vi "MEASURE_2dmapping-2.vi"() -> ()   [LabVIEW 2020]
uses:
  <vilib>/Math Plots/3D Math Plots/3D Surface/3D Surface XCtrl/3D Surface.xctl
  <vilib>/Math Plots/3D Math Plots/3D Surface/3D Surface Datatype/3D Surface Datatype.lvclass
  <instrlib>/Keithley 24XX/Public/Data/Read (Multiple Points).vi
  <vilib>/Utility/file.llb/Write To Spreadsheet File (DBL).vi
  <vilib>/Math Plots/3D Math Plots/3D Surface/3D Surface Datatype/Public/Plot Helper (Vector).vi
  C/Program Files/National Instruments/LabVIEW 2016/instr.lib/Stanford Research 830/Stanford Research 830.lvlib
  C/Program Files/National Instruments/LabVIEW 2016/instr.lib/Keithley 2450/Keithley 2450.lvlib
  <instrlib>/Keithley 24XX/Keithley 24XX.lvlib
  <vilib>/Analysis/NI_AALBase.lvlib
panel:
  in  "GATE / SD stablization 5":dbl=0.1 format="%#_13g"
  in  "GATE / SD stablization 4":dbl=0.1 format="%#_13g"
  in  "ramping step":i32=20
  in  "Compliance  Level (1uA) 2":dbl=1e-08
  in  "Source Mode  (0: Voltage) 2":u16(ring) items=["Voltage", "Current"]
  out "3D Surface":refnum<class "3D Plot Datatype.lvclass">[](xcontrol)
  in  "scaning step2":i32=60
  out "gate voltage1":dbl=3.0 format="%#_13g"
  in  "scanning step1":i32=30
  in  "GATE2 end Value   2":dbl=10.0
  in  "GATE2 starting Value  2":dbl=-14.0
  out "gate 2leaking":dbl=1.1399661770106206e-10
  out "gate voltage2":dbl=10.0 format="%#_13g"
  in  "Serial Configuration":T1={"Baud Rate"=9600, "Parity"=0, "Data Bits"=8, "Stop Bits"=10, "Flow Control"=0} {"Flow Control" items=["None", "XON/XOFF", "RTS/CTS", "XON/XOFF & RTS/CTS", "DTR/DSR", "XON/XOFF & DTR/DSR"]; "Stop Bits" items=["1.0"=10, "1.5"=15, "2.0"=20]; "Data Bits" items=["7"=7, "8"=8]; "Parity" items=["None", "Odd", "Even", "Mark", "Space"]; "Baud Rate" items=["300"=300, "600"=600, "1200"=1200, "2400"=2400, "4800"=4800, "9600"=9600, "19200"=19200]}
  in  "gate2 address":refnum<visa-resource-name>="GPIB0::25::INSTR"
  in  "Save data or not":bool=TRUE
  in  "path (folder + filename)":string="C:\\Users\\User\\Data\\Jason\\03282019\\mapping_3"
  out "XY Graph":cluster{dbl[], dbl[]}(graph)={[-14.0, -13.6, -13.2, -12.8, -12.4, -12.0, -11.6, -11.2, -10.8, -10.4, -10.0, -9.6, -9.2, -8.8, -8.399999999999999, -8.0, -7.6, -7.199999999999999, -6.8, -6.3999999999999995, -6.0, -5.6, -5.199999999999999, -4.799999999999999, -4.399999999999999, -4.0, -3.5999999999999996, -3.1999999999999993, -2.799999999999999, -2.3999999999999986, -2.0, -1.5999999999999996, -1.1999999999999993, -0.7999999999999989, -0.3999999999999986, 0.0, 0.40000000000000036, 0.8000000000000007, 1.200000000000001, 1.6000000000000014, 2.0, 2.400000000000002, 2.8000000000000007, 3.1999999999999993, 3.6000000000000014, 4.0, 4.400000000000002, 4.800000000000001, 5.200000000000003, 5.600000000000001, 6.0, 6.400000000000002, 6.800000000000001, 7.200000000000003, 7.600000000000001, 8.0, 8.400000000000002, 8.8, 9.200000000000003, 9.600000000000001, 10.0], [0.000948314, 0.000947837, 0.000947598, 0.000947479, 0.000947241, 0.000946883, 0.000946645, 0.000945572, 0.000944141, 0.000942711, 0.000941519, 0.000939969, 0.000938658, 0.000937108, 0.00093532, 0.000933651, 0.000931863, 0.000929955, 0.000928048, 0.000926021, 0.000923995, 0.00092173, 0.000919465, 0.0009172, 0.000914697, 0.000912312, 0.000909809, 0.000907306, 0.000904683, 0.00090218, 0.000899557, 0.000896934, 0.000894193, 0.00089157, 0.000888947, 0.000886325, 0.000883702, 0.00088108, 0.000878457, 0.000875834, 0.000873331, 0.000870828, 0.000868324, 0.00086594, 0.000863437, 0.000861172, 0.000858787, 0.000856522, 0.000854257, 0.000852112, 0.000849966, 0.000847939, 0.000846032, 0.000844125, 0.000842217, 0.000840429, 0.000838879, 0.000837211, 0.000835661, 0.00083435, 0.000833277]}
  out "LOCKIN Measurement":dbl=0.000833277
  in  "Parameter (1: X)":u16(ring)=1 items=["X"=1, "Y"=2, "R"=3, "Theta"=4, "Channel 1"=5, "Channel 2"=6, "Aux In 1"=7, "Aux In 2"=8, "Aux In 3"=9, "Aux In 4"=10]
  out "gate leaking":string="4.458176E-12\n"
  in  "GATE1 end Value (default 0)":dbl=3.0
  in  "GATE1 starting(small) Value":dbl=-3.0
  in  "Function (0: Volts) 2":u16(ring) items=["Volts", "Current", "Resistance"]
  in  "Source Compaliance":dbl=1e-08
  in  "gate1 address":refnum<visa-resource-name>="GPIB0::18::INSTR"
  in  "SD stabilization(S) 2":dbl=0.1 format="%#_13g"
  in  "Sine Output Amplitude (1 V) 2":dbl=0.05
  in  "GATE / SD stablization 3":dbl=0.2 format="%#_13g"
  in  "frequency":dbl=50.0 format="%#_13g"
  in  "Input Connection (0: Single-Ended Voltage)":u16(ring) items=["Single-Ended Voltage", "Differential Voltage", "1 MOhm Current Gain", "100 MOhm Current Gain"]
  in  "LOCKIN address":refnum<visa-resource-name>="GPIB0::8::INSTR"
  # "Lock-in"
  # "2450 Gate Setting"
  # "2401 Gate Setting"
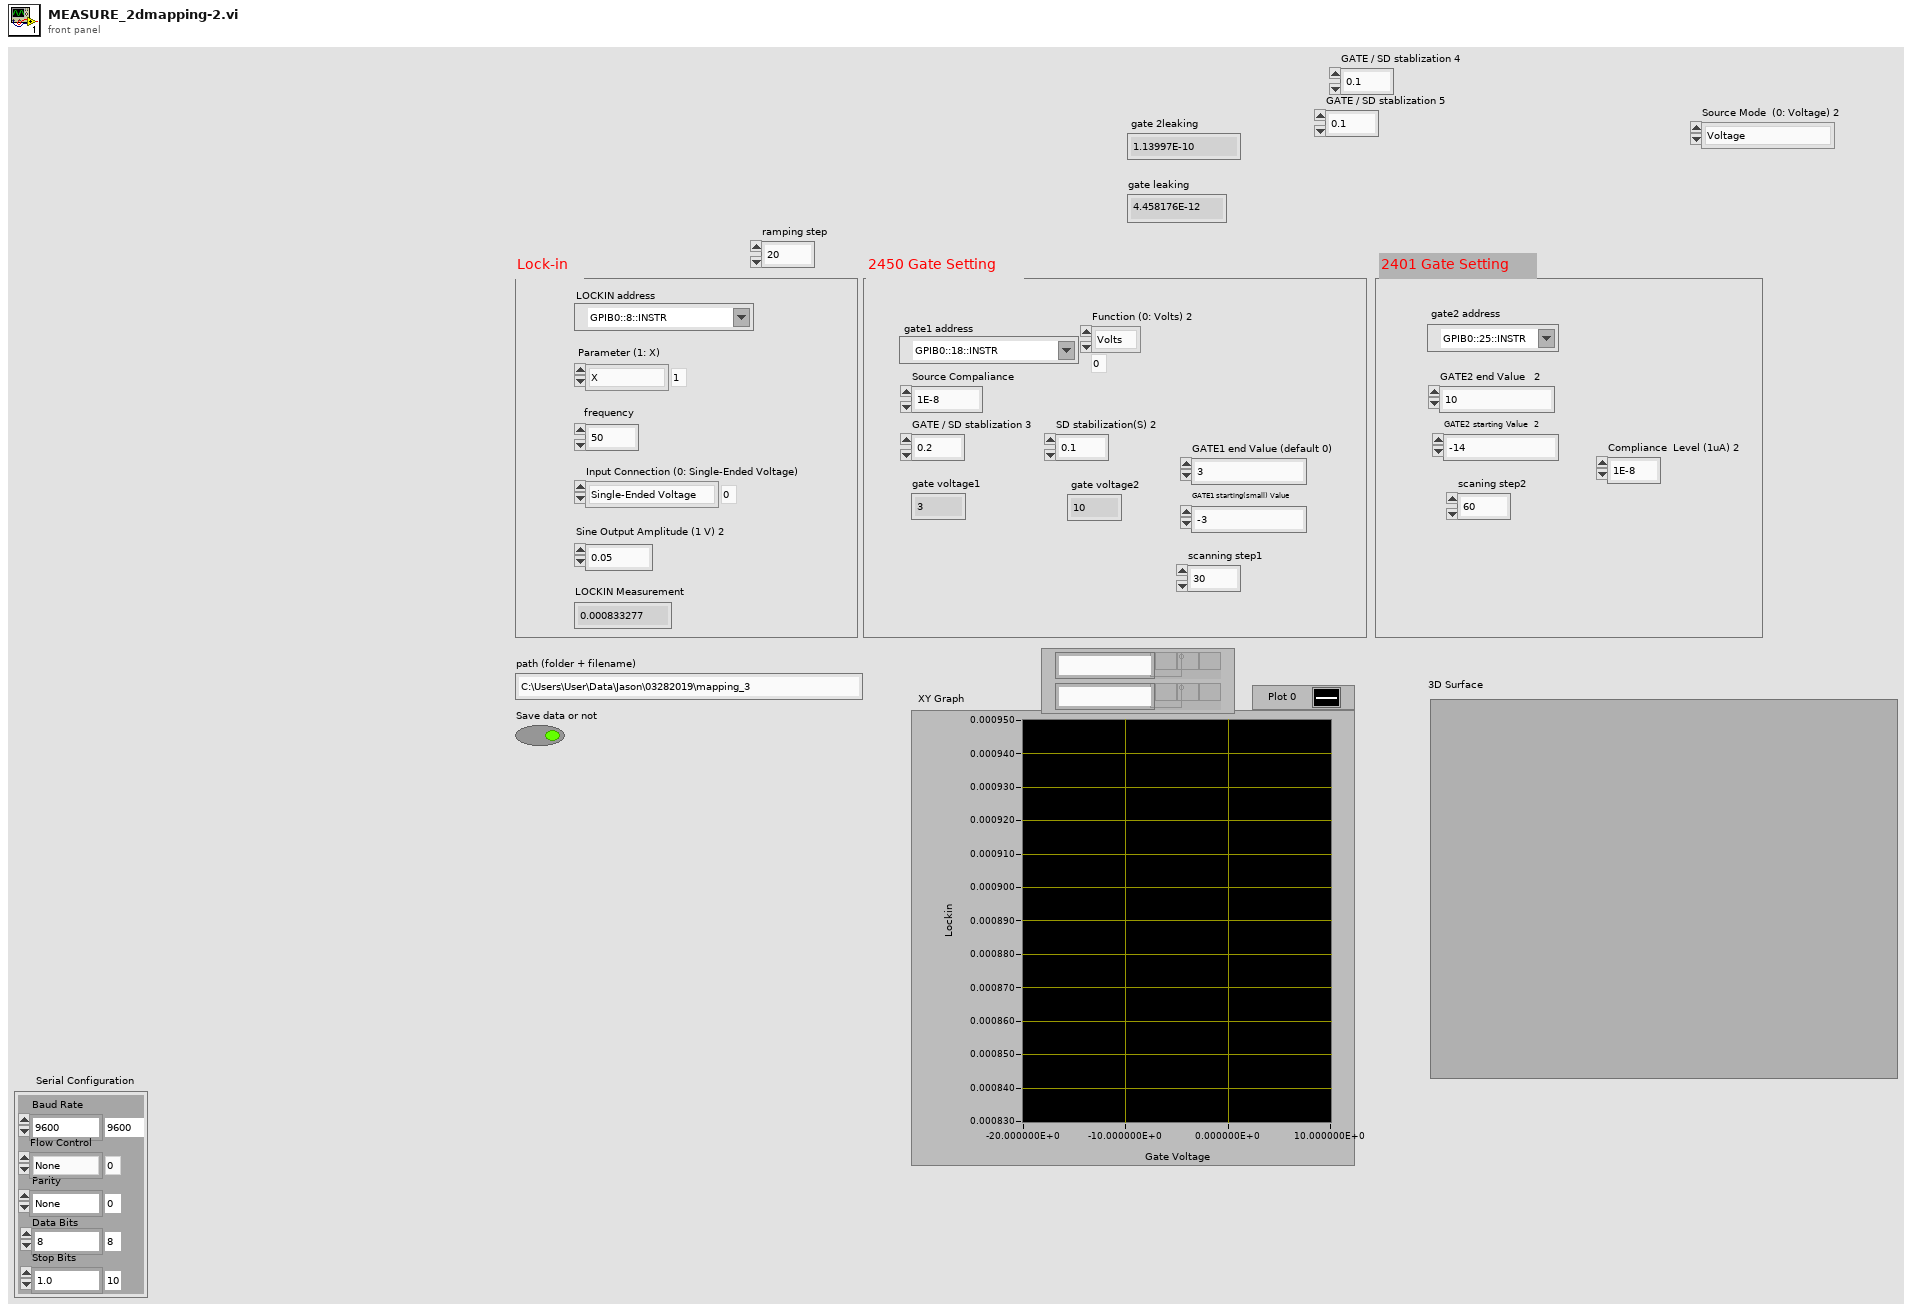
[diagram p1: front panel]
types:
  T1 = cluster{"Baud Rate":u32, "Parity":u16, "Data Bits":u16, "Stop Bits":u16, "Flow Control":u16}
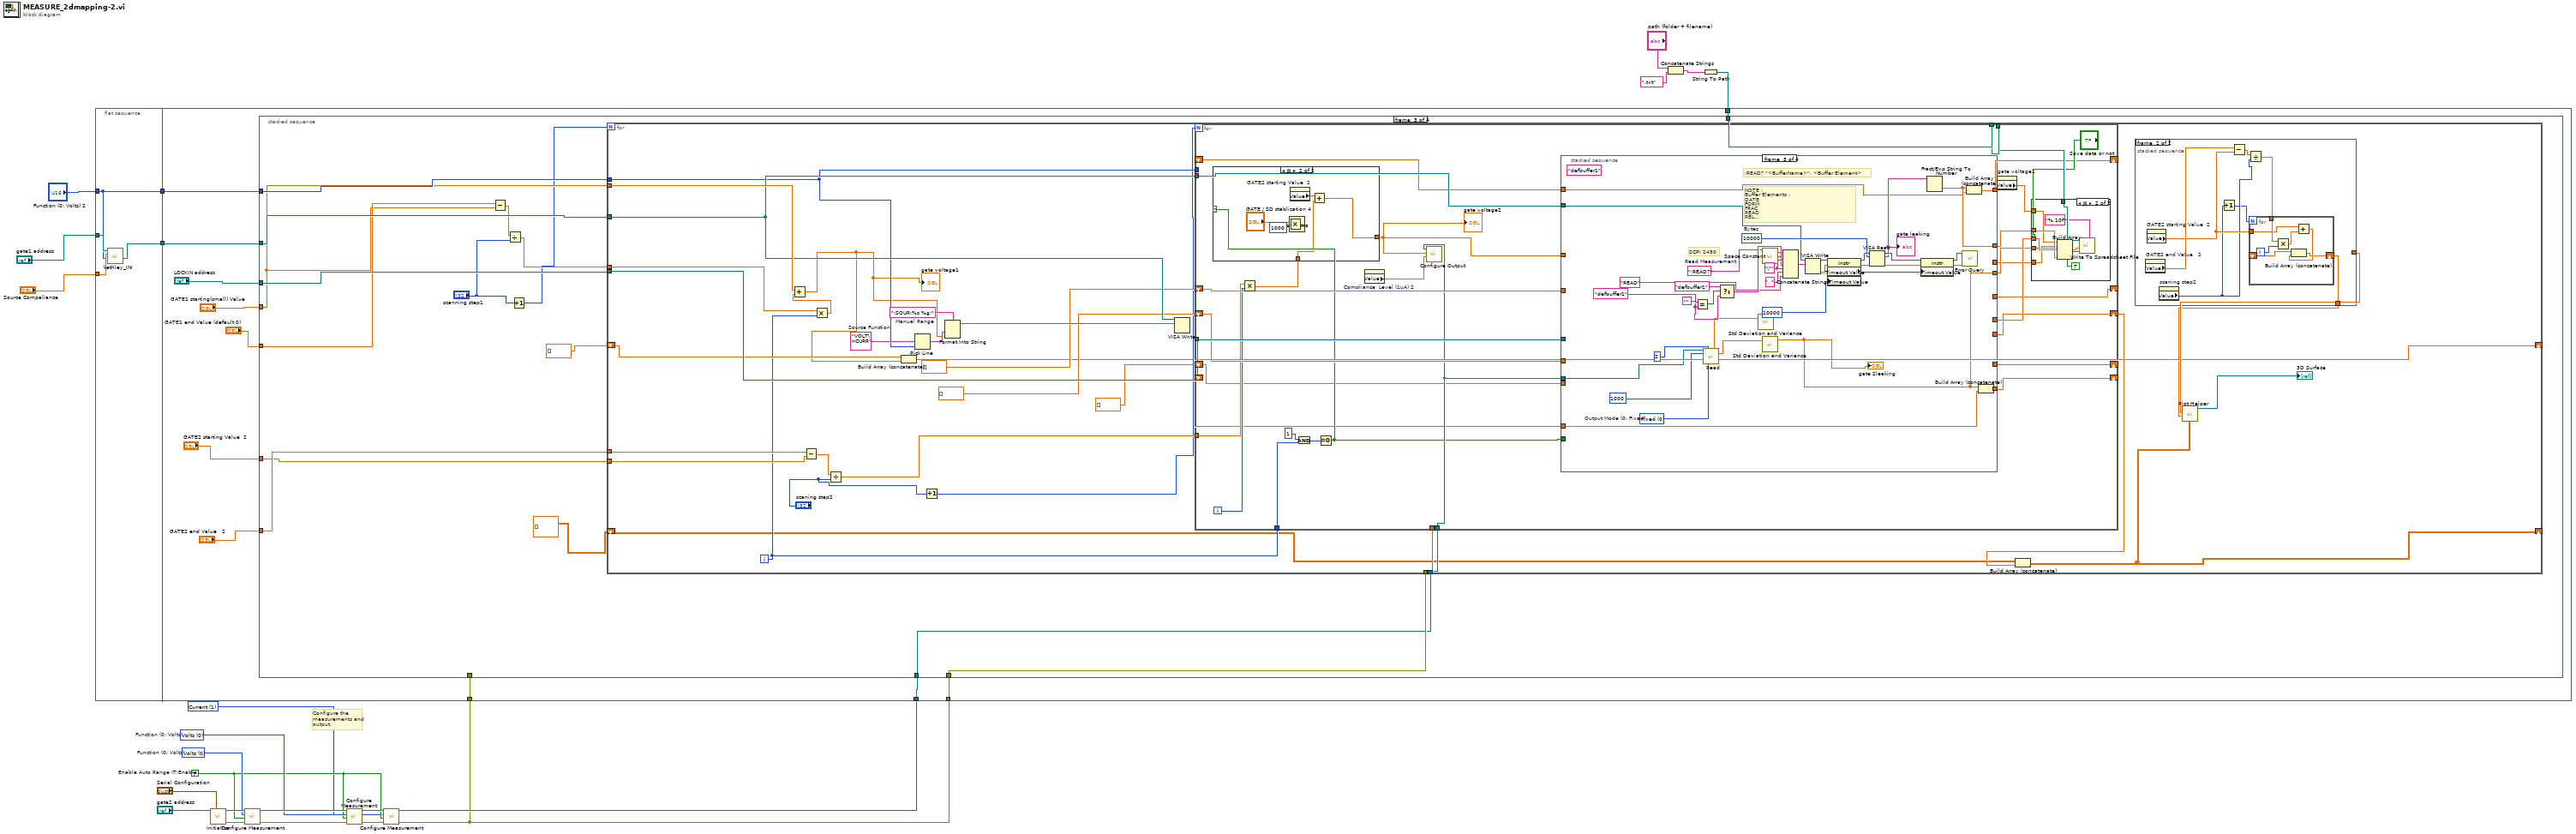
[diagram p0: block diagram]
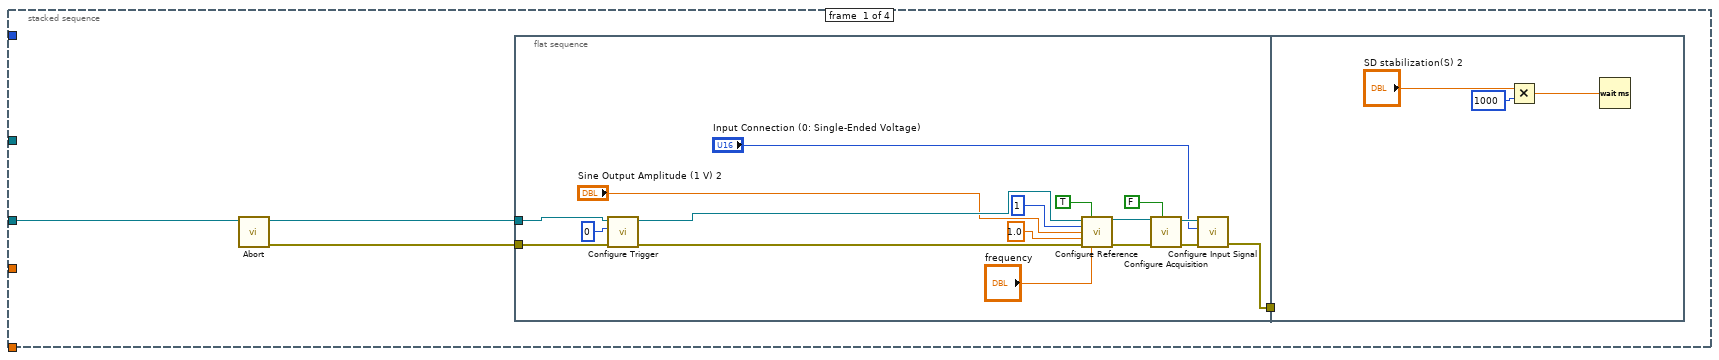
[diagram p2: hidden frame]
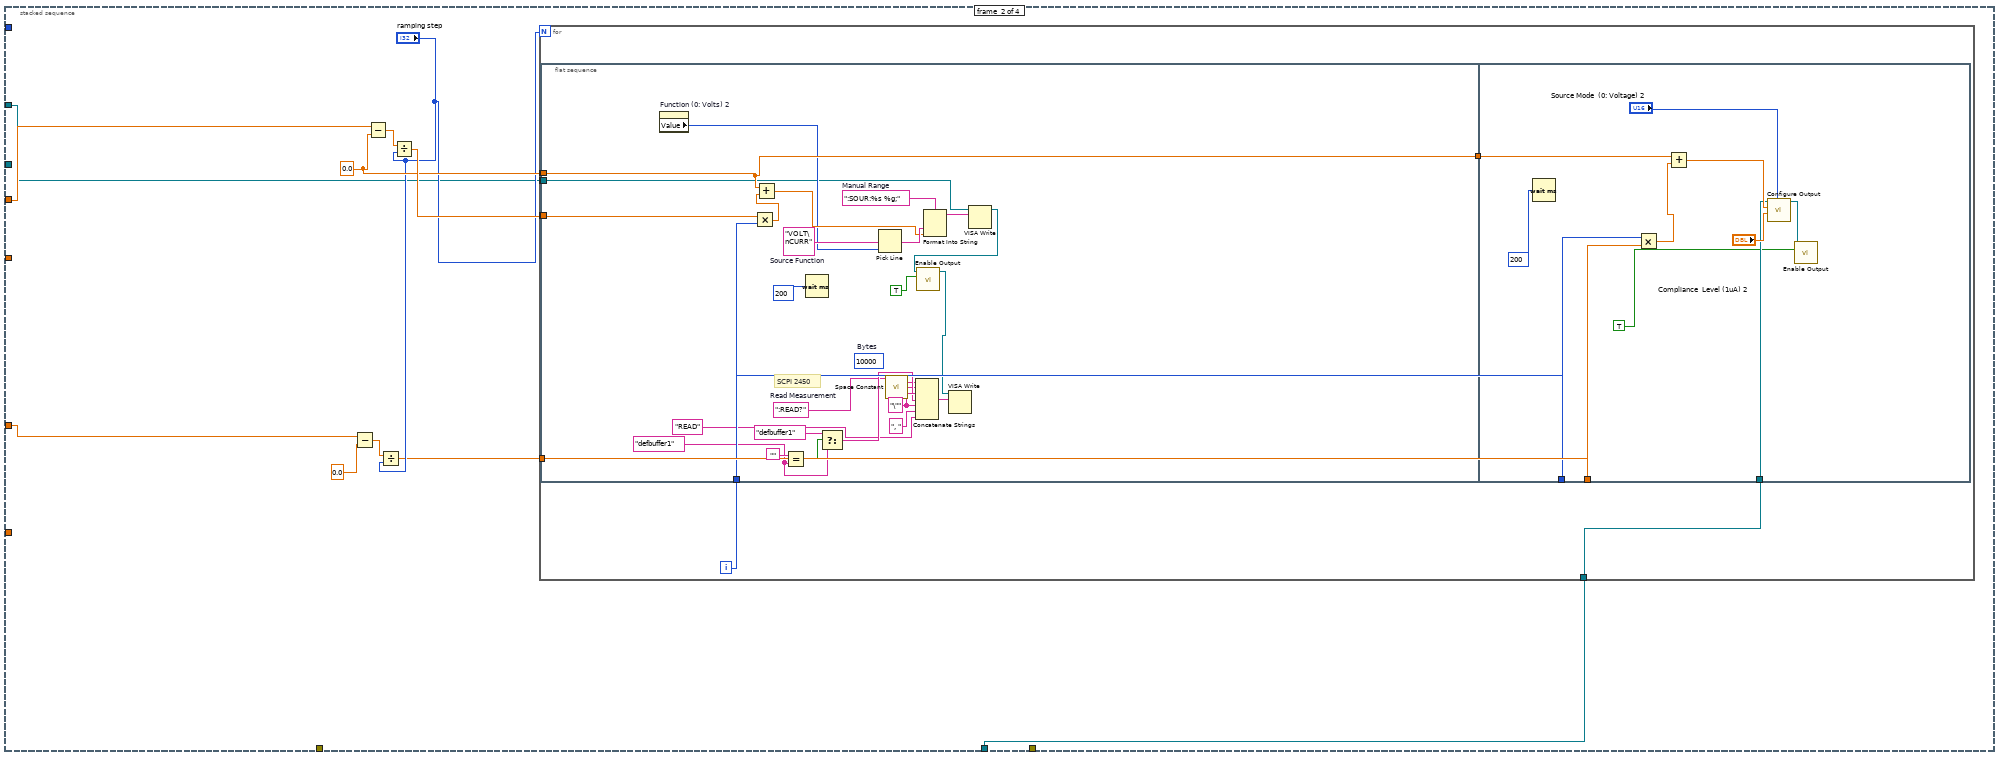
[diagram p3: hidden frame]
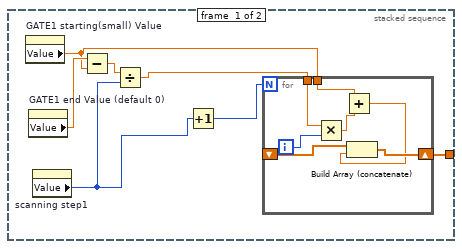
[diagram p4: hidden frame]
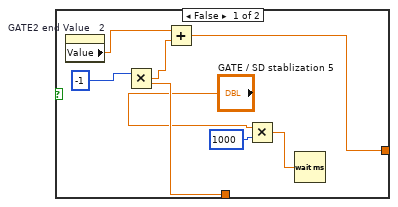
[diagram p5: hidden frame]
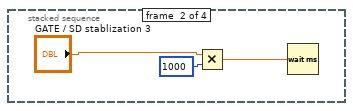
[diagram p8: hidden frame]
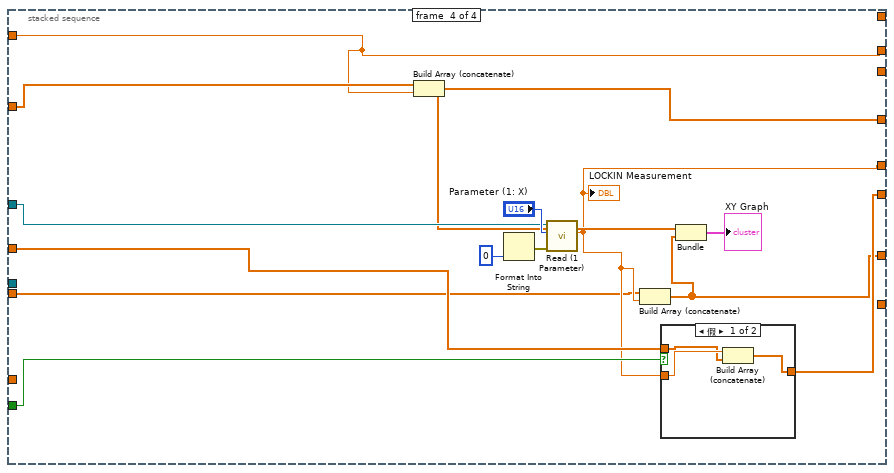
[diagram p9: hidden frame]
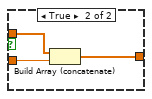
[diagram p10: hidden frame]
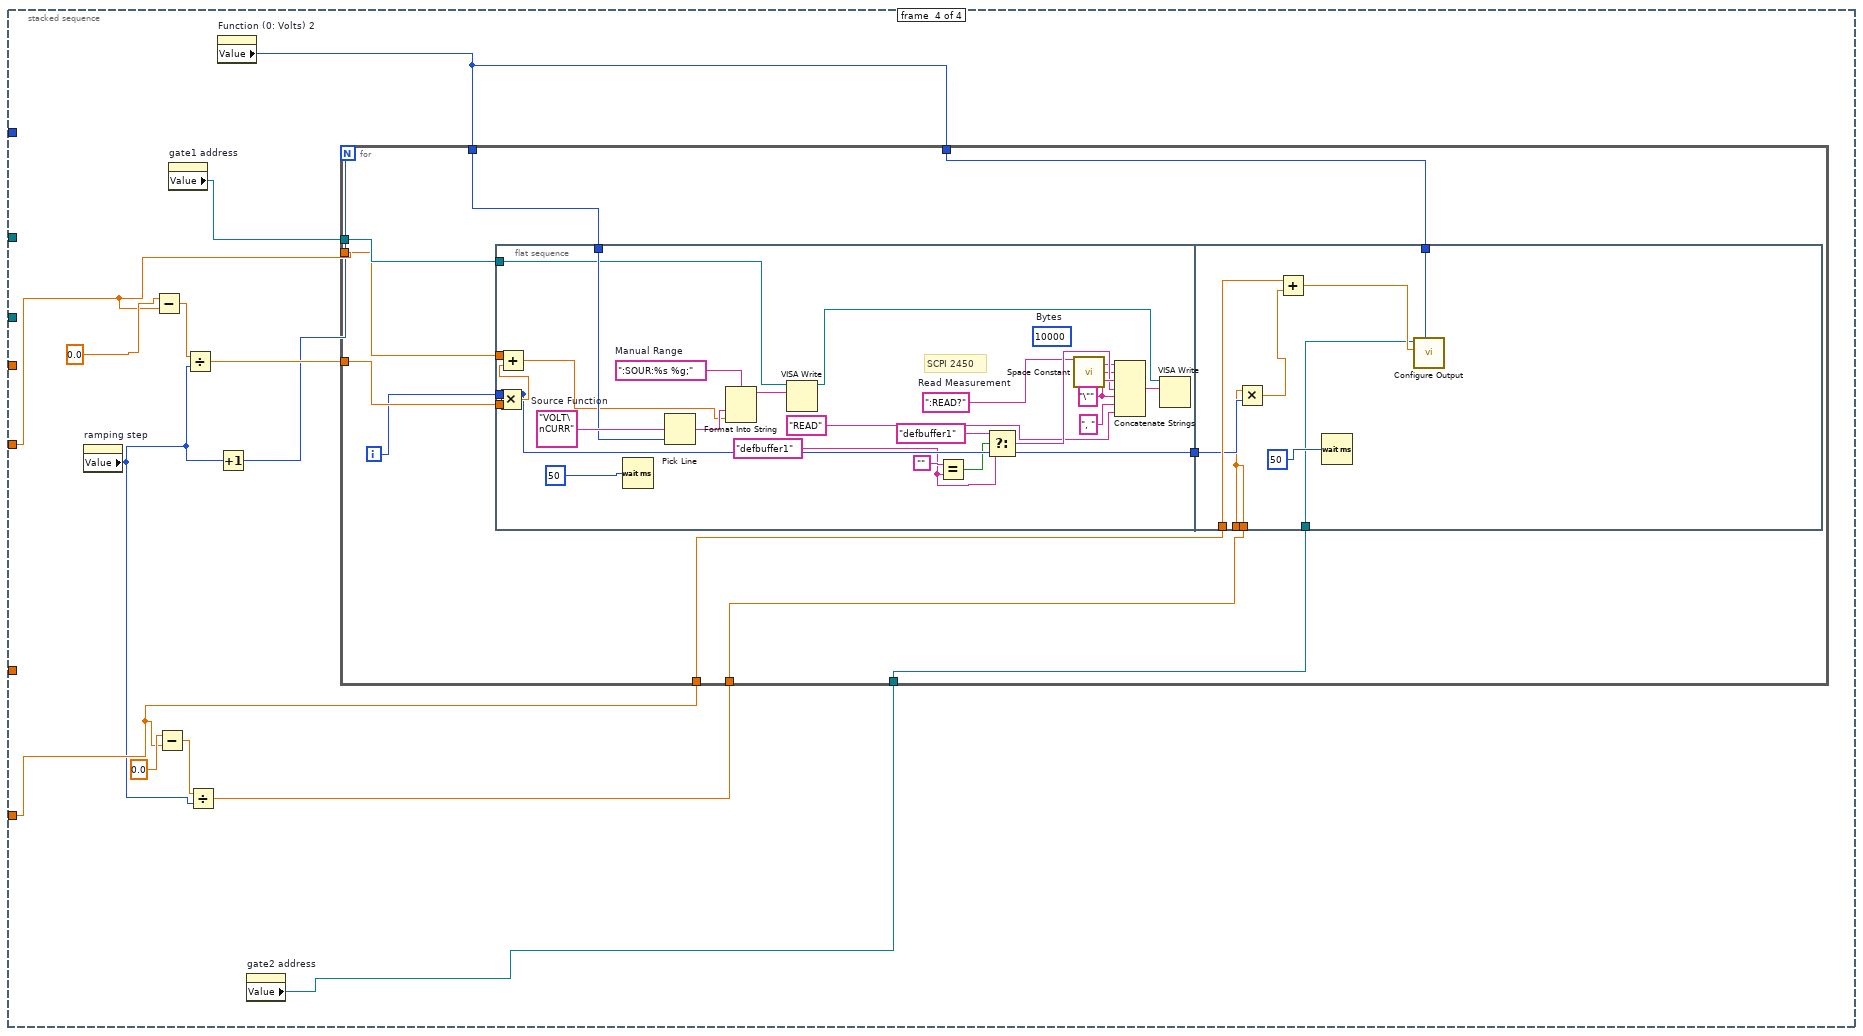
[diagram p11: hidden frame]
diagram:
  w3 = u16 1 items=["Volts", "Current", "Resistance"] ("Function (0: Volts)")
  w4 = TRUE  # Enable Auto Range (T:Enable)
  w7 = u16 0 items=["Volts", "Current", "Resistance"]  # Function (0: Volts)
  w8 = u16 0 items=["Volts", "Current", "Resistance"]  # Function (0: Volts)
  # "Configure the measurements and output."
  n1 = flat-sequence {
    tunnel: "gate1 address" -> [w27]
    tunnel: "Source Compaliance" -> [w26]
    tunnel: "Function (0: Volts) 2" -> [w24]
    tunnel: [w25] -> w20
    tunnel: [w24] -> w19
    tunnel: w20 -> [w37]
    tunnel: w19 -> [w36]
    tunnel: w15 -> [w33]
    tunnel: w2 -> [w32]
    tunnel: w1 -> [w31]
    tunnel: w1 -> [w28]
    frame #0 {
      n2 = call "kethley_INI.vi"("Function (0: Volts) in"=w24, "Source Compaliance"=w26, "VISA Refnum in"=w27) -> ("VISA resource name out"=w25:refnum<visa-resource-name>)  [unwired: 8 in]
    }
    frame #1 {
      n3 = stacked-sequence {
        tunnel: "LOCKIN address" -> [w41 _ w133 _]
        tunnel: w37 -> [_ w64 w130 _]
        tunnel: w36 -> [_ _ w129 _]
        tunnel: "GATE1 starting(small) Value" -> [_ w71 w123 _]
        tunnel: "GATE1 end Value (default 0)" -> [_ _ w124 w309]
        tunnel: w33 -> [_ _ w132 _]
        tunnel: w32 -> [_ w63 w128 _]
        tunnel: w31 -> [_ _ w131 _]
        tunnel: "GATE2 starting Value  2" -> [_ w66 w121 _]
        tunnel: "GATE2 end Value   2" -> [_ _ w122 w307]
        tunnel: w28 -> [_ _ _ _]
        frame #0 {
          n4 = call "Abort.vi"("VISA resource name"=w41) -> ("error out"=w39:errorcluster, "VISA resource name out"=w40:refnum<visa-resource-name>)  [unwired: 9 in]
          n5 = flat-sequence {
            tunnel: w40 -> [w59]
            tunnel: [w44] -> w42
            tunnel: w39 -> [w43]
            tunnel: w42 -> [_]
            frame #0 {
              n6 = call "Configure Trigger.vi"("error in (no error)"=w43, "Trigger Source (0: Internal)"=0, "VISA resource name"=w59) -> ("error out"=w53:errorcluster, "VISA resource name out"=w54:refnum<visa-resource-name>)  [unwired: 7 in]
              n7 = call "Configure Reference.vi"("VISA resource name"=w54, "Auto Phase (T: Enabled)"=TRUE, "Reference Source (1: Internal)"=1, "Sine Output Amplitude (1 V)"="Sine Output Amplitude (1 V) 2", "Detection Harmonic Number (1)"=1.0 ("output voltage 2"), "error in (no error)"=w53, "Internal Reference Frequency (1000 Hz)"="frequency") -> ("VISA resource name out"=w51:refnum<visa-resource-name>, "error out"=w46:errorcluster)  [unwired: 7 in]
              n8 = call "Configure Acquisition.vi"("Continuous Storage (T: Enable)"=FALSE, "error in (no error)"=w46, "VISA resource name"=w51) -> ("error out"=w45:errorcluster, "VISA resource name out"=w49:refnum<visa-resource-name>)  [unwired: 7 in]
              n9 = call "Configure Input Signal.vi"("error in (no error)"=w45, "Input Connection (0: Single-Ended Voltage)"="Input Connection (0: Single-Ended Voltage)", "VISA resource name"=w49) -> ("error out"=w44:errorcluster)  [unwired: 7 in, 1 out]
            }
            frame #1 {
              n10 = Multiply(x="SD stabilization(S) 2", y=1000) -> (x*y=w62:dbl)
              n11 = Wait (ms)(milliseconds to wait=w62) -> ()  [unwired: 1 out]
            }
          }
        }
        frame #1 {
          w70 = 0.0
          n12 = Subtract(x=w66, y=0.0) -> (x-y=w69:dbl)
          n13 = Subtract(x=w71, y=w70) -> (x-y=w73:dbl)
          n14 = Divide(x=w69, y="ramping step") -> (x/y=w65:dbl)
          n15 = Divide(x=w73, y="ramping step") -> (x/y=w72:dbl)
          n16 = for {
            N: "ramping step" -> [_]
            tunnel: w72 -> [w80]
            tunnel: w70 -> [w79]
            tunnel: w65 -> [w78]
            tunnel: w64 -> [w75]
            tunnel: w63 -> [w74]
            i -> [w77]
            n17 = flat-sequence {
              tunnel: w77 -> [w100]
              tunnel: w80 -> [w99]
              tunnel: w79 -> [w98]
              tunnel: [w98] -> w76
              tunnel: w75 -> [w96]
              tunnel: w78 -> [w114]
              tunnel: w77 -> [w113]
              tunnel: w76 -> [w112]
              tunnel: w74 -> [w110]
              frame #0 {
                w81 = "defbuffer1" ("Buffer Name (defbuffer1) 2")
                w89 = "\""
                w86 = ":READ?"  # Read Measurement
                (unwired) u32 10000  # Bytes
                w105 = "VOLT\nCURR"  # Source Function
                w104 = ":SOUR:%s %g;"  # Manual Range
                # "SCPI 2450"
                n18 = property on="Function (0: Volts) 2" class="Ring (严格)"() -> ("Value"=w97:u16)  [unwired: 2 in, 2 out]
                n19 = Multiply(x=w99, y=w100) -> (x*y=w102:dbl)
                n20 = Add(x=w98, y=w102) -> (x+y=w101:dbl)
                n21 = Equal?(x="", y=w81) -> (x = y?=w82:bool)
                n22 = Wait (ms)(milliseconds to wait=200) -> ()  [unwired: 1 out]
                n23 = Select(t="defbuffer1", s=w82, f=w81) -> (s? t:f=w88:string)
                n24 = Pick Line(multi-line string=w105, line index=w97) -> (output string=w106:string)  [unwired: 1 out]
                n25 = call <vilib>:"Space Constant.vi"() -> ("String"=w87:string)
                n26 = Concatenate Strings(w86, w87, w89, w88, w89, ", " ("string"), "READ" ("Buffer Elements 2")) -> (w92:string)
                n27 = Format Into String(format string=w104, w106, w101) -> (resulting string=w103:string)  [unwired: 2 in, 1 out]
                n28 = VISA Write(VISA resource name=w96, write buffer=w103) -> (VISA resource name out=w94:refnum<visa-resource-name>)  [unwired: 1 in, 2 out]
                n29 = call <instrlib>:"Enable Output.vi"("Enable Output (T: Enable)"=TRUE, "VISA resource name"=w94) -> ("VISA resource name out"=w83:refnum<visa-resource-name>)  [unwired: 8 in, 1 out]
                n30 = VISA Write(VISA resource name=w83, write buffer=w92) -> ()  [unwired: 1 in, 3 out]
              }
              frame #1 {
                n31 = Wait (ms)(milliseconds to wait=200) -> ()  [unwired: 1 out]
                n32 = Multiply(x=w113, y=w114) -> (x*y=w115:dbl)
                n33 = Add(x=w112, y=w115) -> (x+y=w116:dbl)
                n34 = call <instrlib>:"Configure Output.vi"("Source Mode  (0: Voltage)"="Source Mode  (0: Voltage) 2", "Compliance  Level (0.1)"="Compliance  Level (1uA) 2", "Output Level (0)"=w116, "VISA resource name"=w110) -> ("VISA resource name out"=w107:refnum<visa-resource-name>)  [unwired: 6 in, 1 out]
                n35 = call <instrlib>:"Enable Output.vi"("Enable Output (T: Enable)"=TRUE, "VISA resource name"=w107) -> ()  [unwired: 8 in, 2 out]
              }
            }
          }
        }
        frame #2 {
          n36 = Subtract(x=w124, y=w123) -> (x-y=w127:dbl)
          n37 = Divide(x=w127, y="scanning step1") -> (x/y=w126:dbl)
          n38 = Increment(x="scanning step1") -> (x+1=w119:i32)
          n39 = for {
            N: w119 -> [_]
            tunnel: w129 -> [w153]
            tunnel: w130 -> [w154]
            tunnel: w133 -> [w165]
            tunnel: w132 -> [w164]
            tunnel: w131 -> [w163]
            tunnel: w128 -> [w162]
            tunnel: w123 -> [w161]
            tunnel: w126 -> [w160]
            shift-right: [w136] -> _
            shift-left: dbl[] [] ("appended array") -> [w148]
            tunnel: w122 -> [w145]
            tunnel: w121 -> [w144]
            shift-right: [w137] -> _
            shift-left: dbl[][] [] ("Intensity Graph") -> [w138]
            i -> [w141]
            w156 = "VOLT\nCURR"  # Source Function
            w157 = ":SOUR:%s %g;"  # Manual Range
            n40 = Subtract(x=w145, y=w144) -> (x-y=w152:dbl)
            n41 = Multiply(x=w160, y=w141) -> (x*y=w159:dbl)
            n42 = Add(x=w161, y=w159) -> (x+y=w147:dbl)
            "gate voltage1" <- w147
            n43 = Divide(x=w152, y="scaning step2") -> (x/y=w151:dbl)
            n44 = Build Array (concatenate)(w148, w147) -> (w136:dbl[])
            n45 = Pick Line(multi-line string=w156, line index=w153) -> (output string=w155:string)  [unwired: 1 out]
            n46 = Increment(x="scaning step2") -> (x+1=w142:i32)
            n47 = Format Into String(format string=w157, w155, w147) -> (resulting string=w158:string)  [unwired: 2 in, 1 out]
            n48 = VISA Write(VISA resource name=w154, write buffer=w158) -> ()  [unwired: 1 in, 3 out]
            n49 = for {
              N: w142 -> [_]
              tunnel: w153 -> [_]
              tunnel: w154 -> [w222]
              tunnel: w165 -> [w221]
              tunnel: w164 -> [w218]
              tunnel: w163 -> [_]
              tunnel: w162 -> [w206]
              shift-right: [w209] -> _
              shift-left: _ -> [w196]
              tunnel: w151 -> [w215]
              shift-right: [w211] -> w146
              shift-left: dbl[] [] ("appended array") -> [w212]
              shift-right: [w199] -> _
              shift-left: dbl[] [] ("appended array") -> [w210]
              shift-right: [w205] -> _
              shift-left: _ -> [w204]
              tunnel: w141 -> [w200]
              shift-right: [w197] -> _
              shift-left: dbl[] [] ("appended array") -> [w195]
              i -> [w202]
              n50 = Multiply(x=w215, y=w202) -> (x*y=w214:dbl)
              n51 = And(x=1, y=w200) -> (x .and. y?=w201:i32)
              n52 = Equal To 0?(x=w201) -> (x = 0?=w198:bool)
              n53 = case shown="真" w198 {
                tunnel: w214 -> [w230 w231]
                tunnel: [w226 w235] -> w213
                frame False {
                  n54 = property on="GATE2 end Value   2" class="DigNum (严格)"() -> ("Value"=w227:dbl)  [unwired: 2 in, 2 out]
                  n55 = Multiply(x=-1, y=w230) -> (x*y=w228:dbl)
                  n56 = Add(x=w227, y=w228) -> (x+y=w226:dbl)
                  n57 = Multiply(x="GATE / SD stablization 5", y=1000) -> (x*y=w225:dbl)
                  n58 = Wait (ms)(milliseconds to wait=w225) -> ()  [unwired: 1 out]
                }
                frame True {
                  n59 = Multiply(x="GATE / SD stablization 4", y=1000) -> (x*y=w234:dbl)
                  n60 = Wait (ms)(milliseconds to wait=w234) -> ()  [unwired: 1 out]
                  n61 = property on="GATE2 starting Value  2" class="DigNum (严格)"() -> ("Value"=w236:dbl)  [unwired: 2 in, 2 out]
                  n62 = Add(x=w236, y=w231) -> (x+y=w235:dbl)
                }
              }
              "gate voltage2" <- w213
              n63 = property on="Compliance  Level (1uA) 2" class="DigNum (严格)"() -> ("Value"=w194:dbl)  [unwired: 2 in, 2 out]
              n64 = call <instrlib>:"Configure Output.vi"("Compliance  Level (0.1)"=w194, "Output Level (0)"=w213, "VISA resource name"=w206) -> ()  [unwired: 7 in, 2 out]
              n65 = stacked-sequence {
                tunnel: w222 -> [_ _ w262 _]
                tunnel: w221 -> [_ _ _ w295]
                tunnel: [_ _ w261 _] -> w205
                tunnel: w212 -> [_ _ _ w290]
                tunnel: [_ _ _ w289] -> w211
                tunnel: [_ _ _ w293] -> w199
                tunnel: [_ _ _ w287] -> w220
                tunnel: [_ _ w259 _] -> w219
                tunnel: [_ _ w253 _] -> w209
                tunnel: w196 -> [_ _ w252 _]
                tunnel: [_ _ w251 _] -> w216
                tunnel: w213 -> [_ _ _ w291]
                tunnel: w210 -> [_ _ _ w292]
                tunnel: [_ _ _ w291] -> w208
                tunnel: w206 -> [_ _ w249 _]
                tunnel: w204 -> [_ _ w250 _]
                tunnel: w198 -> [_ _ _ w288]
                tunnel: [_ _ _ w285] -> w197
                tunnel: w195 -> [_ _ _ w286]
                frame #0 {
                }
                frame #1 {
                  n66 = Multiply(x="GATE / SD stablization 3", y=1000) -> (x*y=w248:dbl)
                  n67 = Wait (ms)(milliseconds to wait=w248) -> ()  [unwired: 1 out]
                }
                frame #2 {
                  w256 = u16 0 items=["Fixed", "Sweep", "List"]  # Output Mode (0: Fixed)
                  w273 = "defbuffer1" ("Buffer Name (defbuffer1) 2")
                  (unwired) "defbuffer1" ("t")
                  w271 = "\""
                  w268 = ":READ?"  # Read Measurement
                  w277 = u32 10000  # Bytes
                  # "NOTE :\nBuffer Elements :\nDATE\nFORM\nFRAC\nREAD\nREL\nSEC\nSOUR\nSOURFORM\nSOURSTAT\nSOURUNIT\nSTAT\nTIME\nTsT\nUNIT"
                  # ":READ? \"<BufferName>\", <Buffer Element>"
                  # "SCPI 2450"
                  n68 = Equal?(x="", y=w273) -> (x = y?=w274:bool)
                  n69 = call-poly <instrlib>:"Read.vi"("VISA resource name"=w249, "Sample Count (1)"=u32 2 ("Number of Samples"), "Timeout (10000 ms)"=1000, "Output Mode (0: Fixed)"=w256) -> ("Voltage"=w254:sgl[], "Current"=w255:sgl[])  [unwired: 5 in, 5 out]
                  n70 = Select(t="defbuffer1", s=w274, f=w273) -> (s? t:f=w270:string)
                  n71 = call <vilib>:"Std Deviation and Variance.vi"("X"=w254) -> ()  [unwired: 1 in, 3 out]
                  n72 = call <vilib>:"Space Constant.vi"() -> ("String"=w269:string)
                  n73 = call <vilib>:"Std Deviation and Variance.vi"("X"=w255) -> ("mean"=w251:dbl)  [unwired: 1 in, 2 out]
                  "gate 2leaking" <- w251
                  n74 = Concatenate Strings(w268, w269, w271, w270, w271, ", " ("string"), "READ" ("Buffer Elements 2")) -> (w284:string)
                  n75 = VISA Write(VISA resource name=w262, write buffer=w284) -> (VISA resource name out=w276:refnum<visa-resource-name>, error out=w283:errorcluster)  [unwired: 1 in, 1 out]
                  n76 = property class="Instr"(reference=w276, error in=w283, "General Settings:Timeout Value"=10000 ("Timeout (10000 ms) 2")) -> (reference out=w282:refnum<visa-resource-name>, error out=w281:errorcluster, "General Settings:Timeout Value"=w278:u32)
                  n77 = VISA Read(VISA resource name=w282, byte count=w277, error in (no error)=w281) -> (VISA resource name out=w280:refnum<visa-resource-name>, read buffer=w260:string, error out=w279:errorcluster)  [unwired: 1 out]
                  "gate leaking" <- w260
                  n78 = property class="Instr"(reference=w280, error in=w279, "General Settings:Timeout Value"=w278) -> (reference out=w266:refnum<visa-resource-name>, error out=w265:errorcluster)
                  n79 = Fract/Exp String To Number(string=w260) -> (number=w259:dbl)  [unwired: 3 in, 1 out]
                  n80 = call "Error Query.vi"("error in (no error)"=w265, "VISA resource name"=w266) -> ()  [unwired: 10 out]
                  n81 = Build Array (concatenate)(w259, w250) -> (w261:dbl[])
                  n82 = Build Array (concatenate)(w251, w252) -> (w253:dbl[])
                }
                frame #3 {
                  n83 = Build Array (concatenate)(w292, w291) -> (w293:dbl[])
                  n84 = Format Into String(0) -> (error out=w298:errorcluster)  [unwired: 3 in, 1 out]
                  n85 = call "Read (1 Parameter).vi"("error in (no error)"=w298, "Parameter (1: X)"="Parameter (1: X)", "VISA resource name"=w295) -> ("Measurement"=w287:dbl)  [unwired: 6 in, 2 out]
                  "LOCKIN Measurement" <- w287
                  n86 = Build Array (concatenate)(w286, w287) -> (w285:dbl[])
                  n87 = case shown="假" w288 {
                    tunnel: w290 -> [w300 w304]
                    tunnel: w287 -> [w301 w303]
                    tunnel: [w299 w302] -> w289
                    frame False {
                      n88 = Build Array (concatenate)(w301, w300) -> (w299:dbl[])
                    }
                    frame True {
                      n89 = Build Array (concatenate)(w304, w303) -> (w302:dbl[])
                    }
                  }
                  n90 = Bundle(w293, w285) -> (→"XY Graph":cluster{dbl[], dbl[]})  [unwired: 1 in]
                }
              }
              n91 = property on="gate voltage1" class="DigNum (严格)"() -> ("Value"=w207:dbl)  [unwired: 2 in, 2 out]
              n92 = case shown="真" "Save data or not" {
                tunnel: w220 -> [_ w245]
                tunnel: w219 -> [_ w244]
                tunnel: w218 -> [_ w242]
                tunnel: w216 -> [_ w239]
                tunnel: w208 -> [_ w238]
                tunnel: w207 -> [_ w237]
                frame False {
                }
                frame True {
                  n93 = Build Array(w237, w238, w245, w239, w244) -> (w243:dbl[])
                  n94 = call-poly <vilib>:"Write To Spreadsheet File.vi"("format (%.3f)"="%.10f", "append to file? (new file:F)"=TRUE, "1D data"=w243, "file path (dialog if empty)"=w242) -> ()  [unwired: 4 in, 1 out]
                }
              }
            }
            n95 = Build Array (concatenate)(w138, w146) -> (w137:dbl[][])
            n96 = stacked-sequence {
              tunnel: [w168 _] -> w139
              tunnel: [_ w182] -> w134
              frame #0 {
                n97 = property on="GATE1 starting(small) Value" class="DigNum (严格)"() -> ("Value"=w169:dbl)  [unwired: 2 in, 2 out]
                n98 = property on="GATE1 end Value (default 0)" class="DigNum (严格)"() -> ("Value"=w172:dbl)  [unwired: 2 in, 2 out]
                n99 = property on="scanning step1" class="DigNum (严格)"() -> ("Value"=w167:i32)  [unwired: 2 in, 2 out]
                n100 = Subtract(x=w172, y=w169) -> (x-y=w171:dbl)
                n101 = Divide(x=w171, y=w167) -> (x/y=w170:dbl)
                n102 = Increment(x=w167) -> (x+1=w166:i32)
                n103 = for {
                  N: w166 -> [_]
                  tunnel: w170 -> [w178]
                  tunnel: w169 -> [w176]
                  shift-right: [w175] -> w168
                  shift-left: _ -> [w174]
                  i -> [w179]
                  n104 = Multiply(x=w178, y=w179) -> (x*y=w177:dbl)
                  n105 = Add(x=w176, y=w177) -> (x+y=w173:dbl)
                  n106 = Build Array (concatenate)(w174, w173) -> (w175:dbl[])
                }
              }
              frame #1 {
                n107 = property on="GATE2 end Value   2" class="DigNum (严格)"() -> ("Value"=w185:dbl)  [unwired: 2 in, 2 out]
                n108 = property on="GATE2 starting Value  2" class="DigNum (严格)"() -> ("Value"=w184:dbl)  [unwired: 2 in, 2 out]
                n109 = property on="scaning step2" class="DigNum (严格)"() -> ("Value"=w181:i32)  [unwired: 2 in, 2 out]
                n110 = Increment(x=w181) -> (x+1=w180:i32)
                n111 = Subtract(x=w185, y=w184) -> (x-y=w183:dbl)
                n112 = Divide(x=w183, y=w181) -> (x/y=w186:dbl)
                n113 = for {
                  N: w180 -> [_]
                  tunnel: w186 -> [w192]
                  shift-right: [w187] -> w182
                  shift-left: _ -> [w190]
                  tunnel: w184 -> [w191]
                  i -> [w193]
                  n114 = Multiply(x=w192, y=w193) -> (x*y=w189:dbl)
                  n115 = Add(x=w191, y=w189) -> (x+y=w188:dbl)
                  n116 = Build Array (concatenate)(w190, w188) -> (w187:dbl[])
                }
              }
            }
            n117 = call-poly <vilib>:"Plot Helper.vi"("z matrix"=w137, "y vector"=w134, "x vector"=w139) -> ("3D Plot lvclass Array out"=→"3D Surface":refnum<class "3D Plot Datatype.lvclass">[])  [unwired: 3 in, 5 out]
          }
        }
        frame #3 {
          n118 = property on="ramping step" class="DigNum (严格)"() -> ("Value"=w306:i32)  [unwired: 2 in, 2 out]
          n119 = Subtract(x=0.0, y=w309) -> (x-y=w316:dbl)
          n120 = Subtract(x=0.0, y=w307) -> (x-y=w314:dbl)
          n121 = property on="gate1 address" class="VISAName"() -> ("Value"=w317:refnum<visa-resource-name>)  [unwired: 2 in, 2 out]
          n122 = Divide(x=w316, y=w306) -> (x/y=w315:dbl)
          n123 = Divide(x=w314, y=w306) -> (x/y=w312:dbl)
          n124 = property on="Function (0: Volts) 2" class="Ring (严格)"() -> ("Value"=w311:u16)  [unwired: 2 in, 2 out]
          n125 = Increment(x=w306) -> (x+1=w305:i32)
          n126 = property on="gate2 address" class="VISAName"() -> ("Value"=w313:refnum<visa-resource-name>)  [unwired: 2 in, 2 out]
          n127 = for {
            N: w305 -> [_]
            tunnel: w311 -> [w327]
            tunnel: w317 -> [w326]
            tunnel: w309 -> [w325]
            tunnel: w315 -> [w324]
            tunnel: w313 -> [w321]
            tunnel: w307 -> [w318]
            tunnel: w312 -> [w319]
            tunnel: w311 -> [w322]
            i -> [w323]
            n128 = flat-sequence {
              tunnel: w327 -> [w346]
              tunnel: w326 -> [w344]
              tunnel: w325 -> [w343]
              tunnel: w324 -> [w342]
              tunnel: w323 -> [w340]
              tunnel: [w340] -> w320
              tunnel: w322 -> [w356]
              tunnel: w321 -> [w355]
              tunnel: w318 -> [w354]
              tunnel: [w352] -> _
              tunnel: w320 -> [w353]
              tunnel: w319 -> [w352]
              frame #0 {
                w328 = "defbuffer1" ("Buffer Name (defbuffer1) 2")
                w336 = "\""
                w333 = ":READ?"  # Read Measurement
                (unwired) u32 10000  # Bytes
                w350 = "VOLT\nCURR"  # Source Function
                w349 = ":SOUR:%s %g;"  # Manual Range
                # "SCPI 2450"
                n129 = Multiply(x=w340, y=w342) -> (x*y=w347:dbl)
                n130 = Add(x=w343, y=w347) -> (x+y=w345:dbl)
                n131 = Wait (ms)(milliseconds to wait=50) -> ()  [unwired: 1 out]
                n132 = Pick Line(multi-line string=w350, line index=w346) -> (output string=w351:string)  [unwired: 1 out]
                n133 = Format Into String(format string=w349, w351, w345) -> (resulting string=w348:string)  [unwired: 2 in, 1 out]
                n134 = VISA Write(VISA resource name=w344, write buffer=w348) -> (VISA resource name out=w329:refnum<visa-resource-name>)  [unwired: 1 in, 2 out]
                n135 = Equal?(x="", y=w328) -> (x = y?=w330:bool)
                n136 = Select(t="defbuffer1", s=w330, f=w328) -> (s? t:f=w335:string)
                n137 = call <vilib>:"Space Constant.vi"() -> ("String"=w334:string)
                n138 = Concatenate Strings(w333, w334, w336, w335, w336, ", " ("string"), "READ" ("Buffer Elements 2")) -> (w339:string)
                n139 = VISA Write(VISA resource name=w329, write buffer=w339) -> ()  [unwired: 1 in, 3 out]
              }
              frame #1 {
                n140 = Multiply(x=w352, y=w353) -> (x*y=w357:dbl)
                n141 = Add(x=w354, y=w357) -> (x+y=w358:dbl)
                n142 = Wait (ms)(milliseconds to wait=50) -> ()  [unwired: 1 out]
                n143 = call <instrlib>:"Configure Output.vi"("Source Mode  (0: Voltage)"=w356, "Output Level (0)"=w358, "VISA resource name"=w355) -> ()  [unwired: 7 in, 2 out]
              }
            }
          }
        }
      }
    }
  }
  n144 = call <instrlib>:"Initialize.vi"("Serial Configuration"="Serial Configuration", "VISA resource name"="gate2 address") -> ("error out"=w13:errorcluster, "VISA resource name out"=w14:refnum<visa-resource-name>)  [unwired: 8 in]
  n145 = call <instrlib>:"Configure Measurement.vi"("error in (no error)"=w13, "Enable Auto Range (T:Enable)"=w4, "Function (0: Volts)"=w8, "VISA resource name"=w14) -> ("error out"=w12:errorcluster, "VISA resource name out"=w11:refnum<visa-resource-name>)  [unwired: 6 in]
  n146 = call <instrlib>:"Configure Measurement.vi"("error in (no error)"=w12, "Enable Auto Range (T:Enable)"=w4, "Function (0: Volts)"=w7, "VISA resource name"=w11) -> ("error out"=w5:errorcluster, "VISA resource name out"=w6:refnum<visa-resource-name>)  [unwired: 6 in]
  n147 = call <instrlib>:"Configure Measurement.vi"("error in (no error)"=w5, "Enable Auto Range (T:Enable)"=w4, "Function (0: Volts)"=w3, "VISA resource name"=w6) -> ("error out"=w1:errorcluster, "VISA resource name out"=w2:refnum<visa-resource-name>)  [unwired: 6 in]
  n148 = Concatenate Strings("path (folder + filename)", ".txt") -> (w16:string)
  n149 = String To Path(string=w16) -> (path=w15:path)
